vi "Test Method Result when Error.vi"(8 "error in (no error)":errorcluster, 11 "Test Assertion Results in":refnum<class "Assertion Result Test.lvclass">) -> (0 "error out":errorcluster, 3 "Test Assertion Results out":refnum<class "Assertion Result Test.lvclass">)   [LabVIEW 2020, in "LUnit Tests.lvlib" / "Assertion Result Test.lvclass"]
uses:
  Assertion Result Test.lvclass
  C:/Program Files (x86)/National Instruments/LabVIEW 2020/vi.lib/Astemes/LUnit/Test Case.lvclass
  Test Dummys/Test Case Test Double/Test Case Test Double.lvclass
  source/Framework/Result Types/Assertion Result/Public/TypeDefs/Status.ctl
  <vilib>/Astemes/LUnit/Test Case.lvclass/Test Case.ctl
  <vilib>/Astemes/LUnit/Palette/Fail.vi
  <vilib>/Astemes/LUnit/Palette/Pass.vi
  <vilib>/Astemes/LUnit/Set Assertion Type.vi
  <vilib>/Astemes/LUnit/Add test result.vi
  <vilib>/Astemes/LUnit/LUnit Record Assertion Result.vi
  <vilib>/Astemes/LUnit/LUnit Aggregate Assertion Results.vi
  <vilib>/Astemes/LUnit/Method Result/LUnit Merge Status.vi
  <vilib>/Astemes/LUnit/LUnit Concatenate result strings.vi
  <vilib>/Astemes/LUnit/Test Case.lvclass
  source/Framework/Result Types/Assertion Result/Assertion Result.lvlib
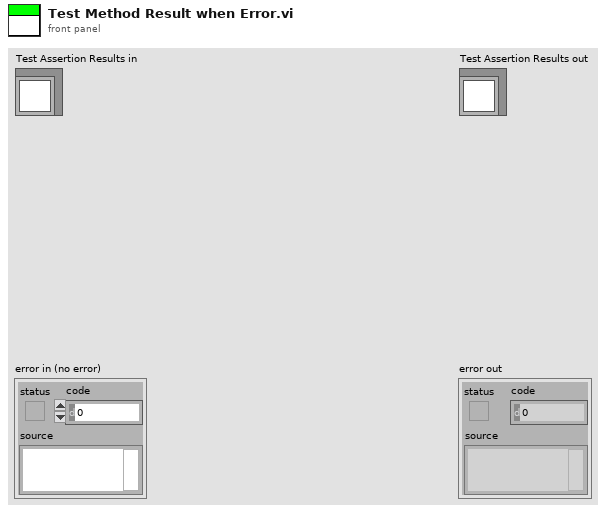
[diagram p1: front panel]
types:
  T1 = typedef "Assertion Result.lvlib/Status.ctl" = enum16{"Pass", "Fail", "Error", "Skipped", "Setup Error", "Broken", "Teardown Error"}
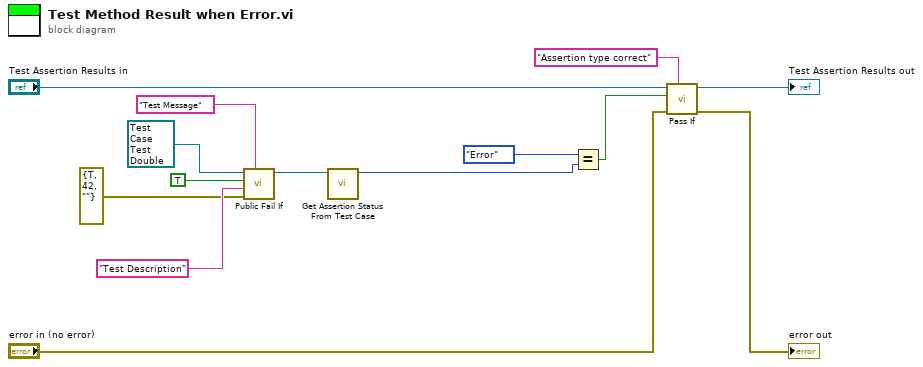
[diagram p0: block diagram]
diagram:
  n1 = call "Public Fail If.vi"("Message"="Test Message", "error in (no error)"=errorcluster {"status"=TRUE, "code"=42, "source"=""}, "Description"="Test Description", "Fail?"=TRUE, "Test Case Test Double in"=refnum<class "Test Case Test Double.lvclass"> refnum ("Test Case Test Double.lvclass")) -> ("Test Case Test Double out"=w13:refnum<class "Test Case Test Double.lvclass">)  [unwired: 5 in, 1 out]
  n2 = call "Get Assertion Status From Test Case.vi"("Test Case Test Double in"=w13) -> ("Status"=w4:T1)  [unwired: 10 in]
  n3 = Equal?(x=Status."Error", y=w4) -> (x = y?=w7:bool)
  n4 = call <vilib>:"Pass If.vi"("Description"="Assertion type correct", "error in (no error)"="error in (no error)", "Pass?"=w7, "LUnit Test Case In"="Test Assertion Results in") -> ("error out"=→"error out":errorcluster, "LUnit Test Case Out"=→"Test Assertion Results out":refnum<class "Assertion Result Test.lvclass">)  [unwired: 6 in]
